vi "Fix path [scalar].vi"(8 "error in (no error)":errorcluster, 10 "Path in":string, 11 "File Transfer Behavior in":refnum<class "File Transfer Behavior.lvclass">) -> (0 "error out":errorcluster, 2 "Path out":string, 3 "File Transfer Behavior out":refnum<class "File Transfer Behavior.lvclass">)   [LabVIEW 2015, in "RT Management.lvlib" / "File Transfer Behavior.lvclass"]
doc: "The path is correctly configured to work in as many situations as possible. Any given path should be returned by this VI in the form \"/path1/path2/path3\", where path1 does not equal \"C\", \"C:\", \"c\", or \"c:\".\n\nFor example, the path \"C:\\blah\\directory\\\" would be transformed to \"/blah/directory\".\n\nThe path in may not contain the characters \"\\\" or \"/\" in their filename. Otherwise, this VI may return an invalid path and/or the path was invalid to begin with."
uses:
  File Transfer Behavior.lvclass
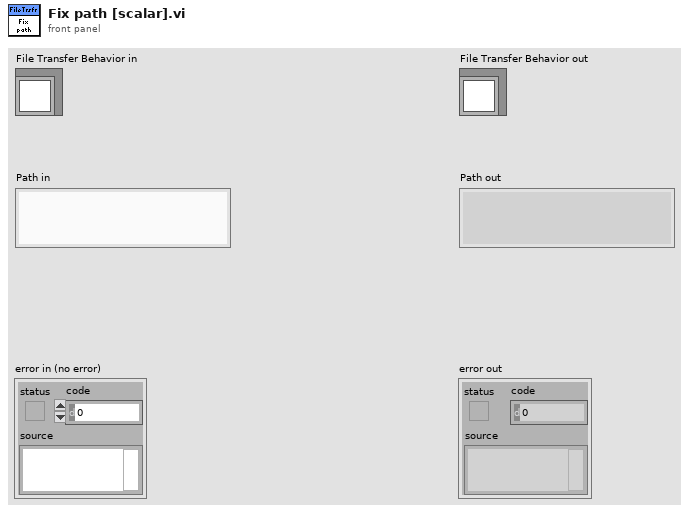
[diagram p1: front panel]
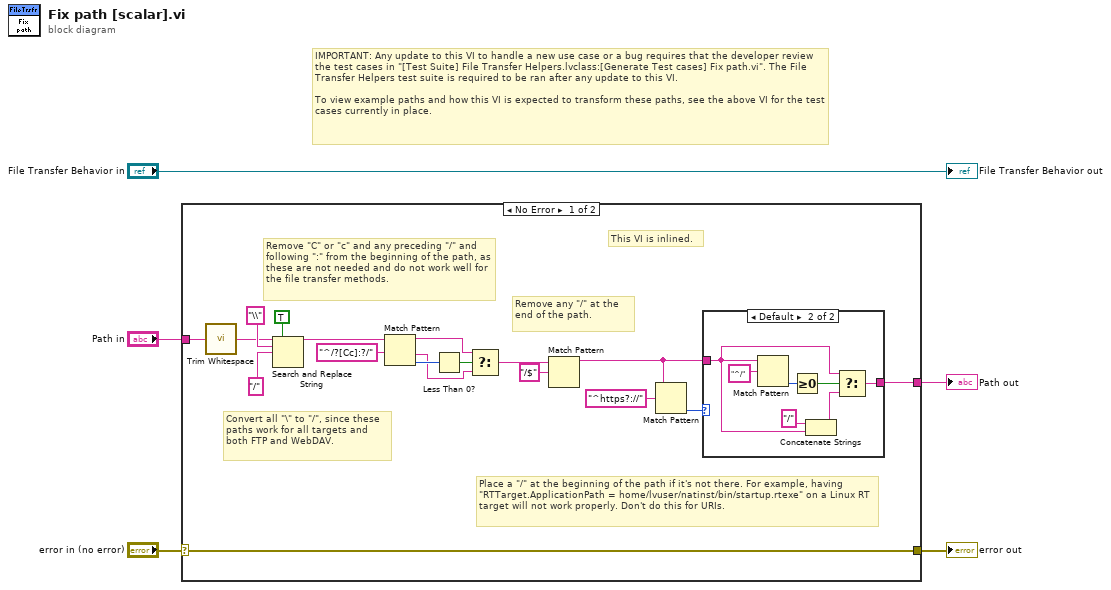
[diagram p0: block diagram]
diagram:
  # "IMPORTANT: Any update to this VI to handle a new use case or a bug requires that the developer review the test cases in \"[Test Suite] File Transfer Helpers.lvclass:[Generate Test cases] Fix path.vi\". The File Transfer Helpers test suite is required to be ran after any update to this VI.\n\nTo view example paths and how this VI is expected to transform these paths, see the above VI for the test cases currently in place."
  n1 = case shown="No Error" "error in (no error)" {
    selector: "error in (no error)" -> [w6 w33]
    tunnel: [w6 w33] -> w4
    tunnel: "Path in" -> [w23 w32]
    tunnel: [w13 w32] -> w2
    frame No Error {
      # "This VI is inlined."
      # "Remove any \"/\" at the end of the path."
      # "Place a \"/\" at the beginning of the path if it's not there. For example, having \"RTTarget.ApplicationPath = home/lvuser/natinst/bin/startup.rtexe\" on a Linux RT target will not work properly. Don't do this for URIs."
      # "Remove \"C\" or \"c\" and any preceding \"/\" and following \":\" from the beginning of the path, as these are not needed and do not work well for the file transfer methods."
      # "Convert all \"\\\" to \"/\", since these paths work for all targets and both FTP and WebDAV."
      n2 = call <vilib>:"Trim Whitespace.vi"("string"=w23) -> ("trimmed string"=w7:string)  [unwired: 1 in]
      n3 = Search and Replace String(replace all?=TRUE ("replace all? (F)"), input string=w7, search string="\\", replace string="/" ("replace string (\"\")")) -> (result string=w12:string)  [unwired: 4 in, 3 out]
      n4 = Match Pattern(string=w12, regular expression="^/?[Cc]:?/") -> (before substring=w18:string, after substring=w16:string, offset past match=w19:i32)  [unwired: 1 in, 1 out]
      n5 = Less Than 0?(x=w19) -> (x < 0?=w17:bool)
      n6 = Select(t=w18, s=w17, f=w16) -> (s? t:f=w8:string)
      n7 = Match Pattern(string=w8, regular expression="/$") -> (before substring=w11:string)  [unwired: 1 in, 3 out]
      n8 = Match Pattern(string=w11, regular expression="^https?://") -> (offset past match=w9:i32)  [unwired: 1 in, 3 out]
      n9 = case shown="Default" w9 {
        tunnel: w11 -> [w24 w27]
        tunnel: [w24 w25] -> w13
        frame 0.. {
        }
        frame Default {
          n10 = Match Pattern(string=w27, regular expression="^/") -> (offset past match=w31:i32)  [unwired: 1 in, 3 out]
          n11 = Greater Or Equal To 0?(x=w31) -> (x >= 0?=w30:bool)
          n12 = Concatenate Strings("/" ("string"), w27) -> (w28:string)
          n13 = Select(t=w27, s=w30, f=w28) -> (s? t:f=w25:string)
        }
      }
    }
    frame Error {
    }
  }
  "error out" <- w4
  "Path out" <- w2
  "File Transfer Behavior out" <- "File Transfer Behavior in"
